vi "daq3 (1).vi"() -> ()   [LabVIEW 2020]
panel:
  in  "array":dbl[](array[numeric])
  out "s? t:f 2":dbl
  in  "stop":bool
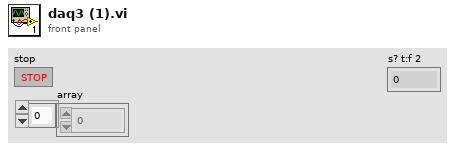
[diagram p1: front panel]
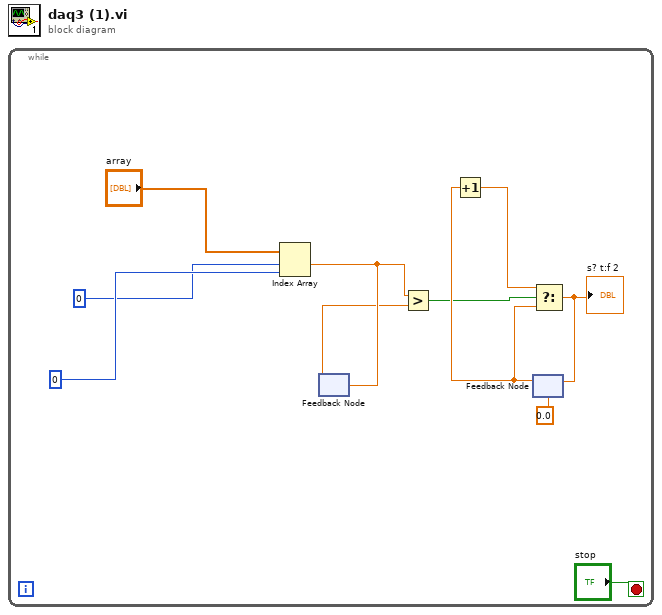
[diagram p0: block diagram]
diagram:
  n1 = while {
    stop <- "stop" stop-if-true
    n2 = Index Array(array="array", index #1=0 ("index"), index #2=0 ("index")) -> (element #1=w3:dbl)  [unwired: 1 out]
    n3 = feedback #1() -> (w2:dbl)  [unwired: 1 in]
    n4 = feedback-in #1(w3) -> ()
    n5 = Greater?(x=w3, y=w2) -> (0:w7:bool)
    n6 = feedback #2(0.0) -> (w8:dbl)
    n7 = Increment(x=w8) -> (x+1=w9:dbl)
    n8 = Select(t=w9, s=w7, f=w8) -> (s? t:f=w5:dbl)
    "s? t:f 2" <- w5
    n9 = feedback-in #2(w5) -> ()
  }
